vi "Toggle Switch.vi"(1 "Input":bool) -> (0 "Output":bool)   [LabVIEW 2014]
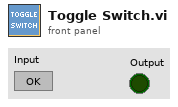
[diagram p1: front panel]
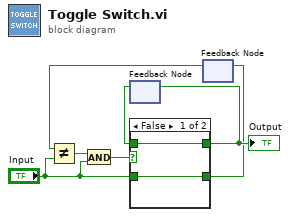
[diagram p0: block diagram]
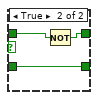
[diagram p2: hidden frame]
diagram:
  n1 = feedback #1() -> (w7:bool)  [unwired: 1 in]
  n2 = feedback #2() -> (w4:bool)  [unwired: 1 in]
  n3 = Not Equal?(x=w4, y="Input") -> (x != y?=w3:bool)
  n4 = And(x=w3, y="Input") -> (x .and. y?=w2:bool)
  n5 = case shown="False" w2 {
    tunnel: w7 -> [w9 w12]
    tunnel: [w9 w11] -> w6
    tunnel: [w8 w10] -> w5
    tunnel: "Input" -> [w8 w10]
    frame False {
    }
    frame True {
      n6 = Not(x=w12) -> (.not. x?=w11:bool)
    }
  }
  "Output" <- w6
  n7 = feedback-in #1(w6) -> ()
  n8 = feedback-in #2(w5) -> ()
